vi "getData.vi"(8 "error in (no error)":errorcluster, 11 "FileReader in":refnum<class "FileReader.lvclass">) -> (0 "error out":errorcluster, 2 "Data":T1, 3 "FileReader out":refnum<class "FileReader.lvclass">)   [LabVIEW 2011, in "Tools.lvlib" / "Filing.lvlib" / "FileReader.lvclass"]
uses:
  FileReader.lvclass
  Hal/Channels/VoltOutput/AnalogOutput.lvclass
  Hal/Channels/Digital/DigitalOutput.lvclass
  Hal/Channels/DDSOutput/Generic/DDSOutput.lvclass
  FileReader.lvclass/FileReader.ctl
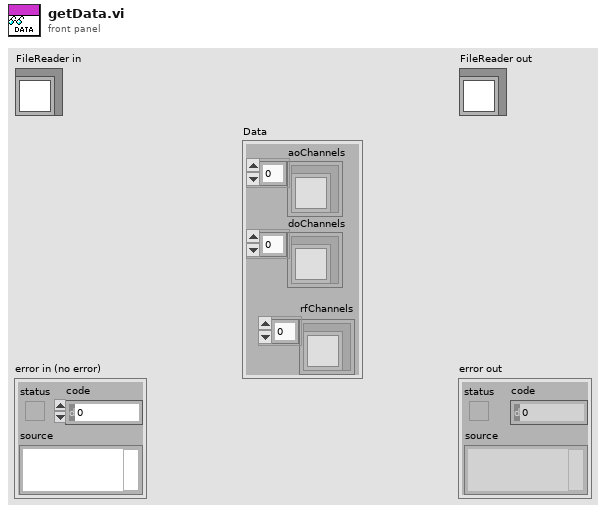
[diagram p1: front panel]
types:
  T1 = cluster{"aoChannels":refnum<class "AnalogOutput.lvclass">[], "doChannels":refnum<class "DigitalOutput.lvclass">[], "rfChannels":refnum<class "DDSOutput.lvclass">[]}
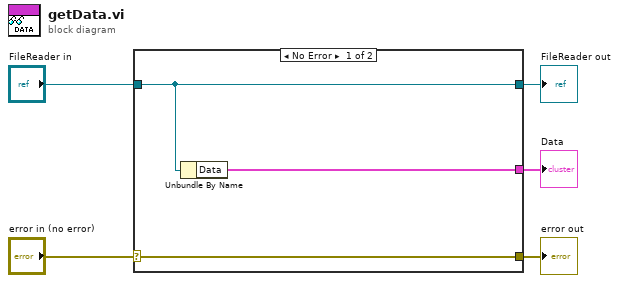
[diagram p0: block diagram]
diagram:
  n1 = case shown="No Error" "error in (no error)" {
    selector: "error in (no error)" -> [w8 w9]
    tunnel: [w8 w9] -> w4
    tunnel: [w7 w10] -> w2
    tunnel: "FileReader in" -> [w7 w10]
    tunnel: [w6 _] -> w1
    frame No Error {
      n2 = Unbundle By Name(w7) -> ("Data"=w6:T1)
    }
    frame Error {
    }
  }
  "error out" <- w4
  "FileReader out" <- w2
  "Data" <- w1
